vi "STM_Server_part_OO.vi"() -> ()   [LabVIEW 2016, in "RemoteControl.STM.lvclass"]
uses:
  RemoteControl.STM.lvclass
  <vilib>/NI/STM/SubVIs/MetaDataElement.ctl
  RemoteControl.STM.lvclass/RemoteControl.STM.ctl
  <vilib>/NI/STM/NI STM.lvlib
panel:
  in  "service name":string
  out "remote address":string
  out "command received":T1
  in  "Enum":T2(ring)
  out "data received":variant
  in  "stop":bool
  out "error out":errorcluster
  # "SERVER  (INSTRUMENT)"
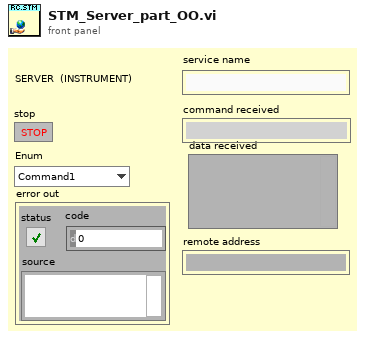
[diagram p1: front panel]
types:
  T1 = typedef "NI STM.lvlib/MetaDataElement.ctl" = string
  T2 = enum16{"Command1", "Command2", "Command3", "Command4", "HELP", "ACK", "CLOSE"}
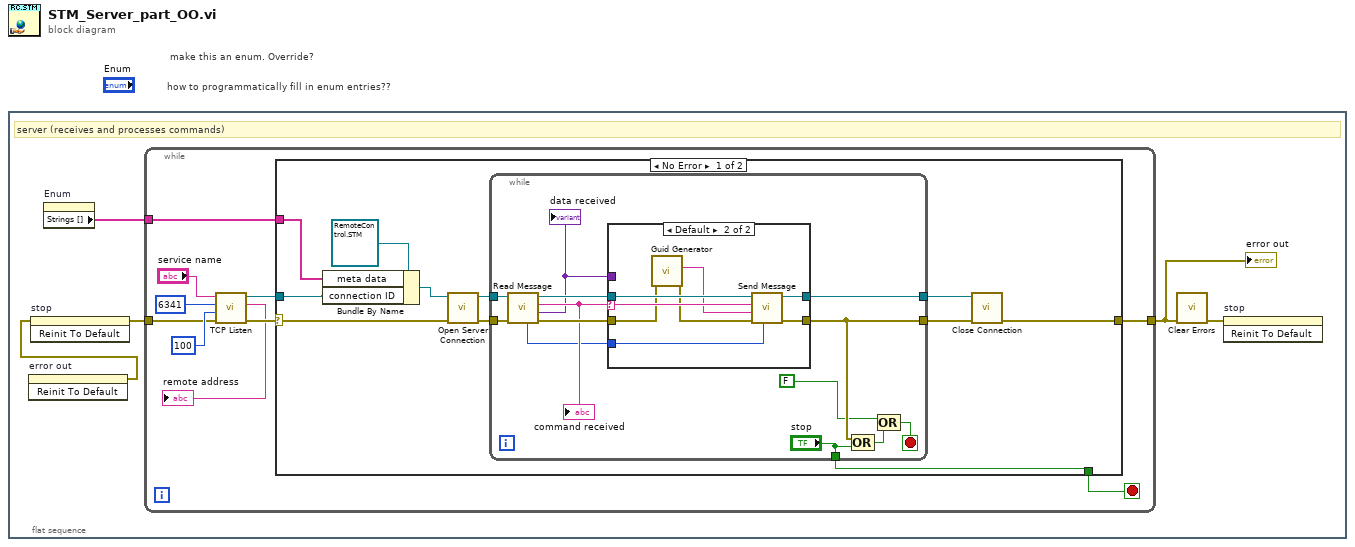
[diagram p0: block diagram]
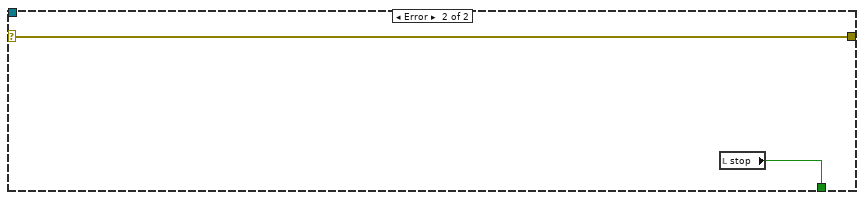
[diagram p3: hidden frame]
diagram:
  # "how to programmatically fill in enum entries??"
  # "make this an enum. Override?"
  n1 = flat-sequence {
    frame #0 {
      # "server (receives and processes commands)"
      n2 = invoke on="error out" class="Clust (strict)" method="Reinit To Default"() -> (error out=w1:errorcluster)  [unwired: 3 in, 2 out]
      n3 = invoke on="stop" class="Bool (strict)" method="Reinit To Default"(error in=w1) -> (error out=w5:errorcluster)  [unwired: 2 in, 2 out]
      n4 = property on="Enum" class="Enum (strict)"() -> ("Strings []"=w2:string[])  [unwired: 2 in, 2 out]
      n5 = while {
        tunnel: w5 -> [w10]
        tunnel: [w9] -> w3
        tunnel: w2 -> [w8]
        stop <- w13 stop-if-true
        n6 = call <vilib>:"TCP Listen.vi"("error in (no error)"=w10, "timeout ms (wait forever: -1)"=100, "port"=u16 6341 ("remote port or service name"), "service name"="service name") -> ("error out"=w11:errorcluster, "remote address"=→"remote address":string, "connection ID"=w14:refnum<k5>)  [unwired: 3 in, 2 out]
        n7 = case shown="No Error" w11 {
          selector: w11 -> [w23 w50]
          tunnel: w14 -> [w24 _]
          tunnel: [w26 w51] -> w13
          tunnel: [w18 w50] -> w9
          tunnel: w8 -> [w16 _]
          frame No Error {
            n8 = Bundle By Name(cluster=refnum<class "RemoteControl.STM.lvclass"> refnum ("RemoteControl.STM in"), "meta data"=w16, "connection ID"=w24) -> (w17:refnum<class "RemoteControl.STM.lvclass">)
            n9 = call-dynamic "Open Server Connection.vi"("error in (no error)"=w23, "RemoteControl.STM in"=w17) -> ("error out"=w22:errorcluster, "RemoteControl.STM out"=w21:refnum<class "RemoteControl.STM.lvclass">)  [unwired: 8 in]
            n10 = while {
              tunnel: [w38] -> w19
              tunnel: [w39] -> w20
              tunnel: ["stop"] -> w26
              tunnel: w22 -> [w33]
              tunnel: w21 -> [w32]
              stop <- w36 stop-if-true
              n11 = call-dynamic "Read Message.vi"("error in (no error)"=w33, "RemoteControl.STM in"=w32) -> ("error out"=w31:errorcluster, "Data"=w27:variant, "Command"=w30:string, "RemoteControl.STM out"=w29:refnum<class "RemoteControl.STM.lvclass">, "Message ID"=w28:i32)  [unwired: 5 in]
              "data received" <- w27
              "command received" <- w30
              n12 = case shown="Default" w30 {
                selector: w30 -> [_ w46]
                tunnel: w29 -> [w40 w47]
                tunnel: [w40 w48] -> w39
                tunnel: w31 -> [w41 w43]
                tunnel: [w41 w49] -> w38
                tunnel: w27 -> [_ _]
                tunnel: w28 -> [_ w45]
                frame "" {
                }
                frame Default {
                  n13 = call <vilib>:"Guid Generator.vi"("error in (no error)"=w43) -> ("error out"=w42:errorcluster, "GUID"=w44:string)  [unwired: 9 in]
                  n14 = call-dynamic "Send Message.vi"("Message ID"=w45, "error in (no error)"=w42, "Data"=w44, "Command"=w46, "RemoteControl.STM in"=w47) -> ("error out"=w49:errorcluster, "RemoteControl.STM out"=w48:refnum<class "RemoteControl.STM.lvclass">)  [unwired: 5 in]
                }
              }
              n15 = Compound Arithmetic op=OR(w38, "stop") -> (w37:bool)
              n16 = Compound Arithmetic op=OR(FALSE ("value"), w37) -> (w36:bool)
            }
            n17 = call-dynamic "Close Connection.vi"("error in (no error)"=w19, "RemoteControl.STM in"=w20) -> ("error out"=w18:errorcluster)  [unwired: 8 in, 1 out]
          }
          frame Error {
            n18 = local read "stop"() -> (w51:bool)
          }
        }
      }
      "error out" <- w3
      n19 = call <vilib>:"Clear Errors.vi"("error in (no error)"=w3) -> ("error out"=w4:errorcluster)  [unwired: 5 in, 1 out]
      n20 = invoke on="stop" class="Bool (strict)" method="Reinit To Default"(error in=w4) -> ()  [unwired: 2 in, 3 out]
    }
  }
